vi "Operator Input Decimal.vi"(7 "Data format":string="0103ddd", 8 "error in (no error)":errorcluster, 9 "Lower limit":dbl=1.0, 10 "Upper limit":dbl=1000000000000000.0, 11 "Message":string) -> (0 "error out":errorcluster, 1 "number":i32, 2 "Stop button hit":bool, 3 "Response":string)   [LabVIEW 2013]
panel:
  in  "stop":bool
  in  "Response1":string
  # "Operator Message"
  # "Scan or Enter Response"
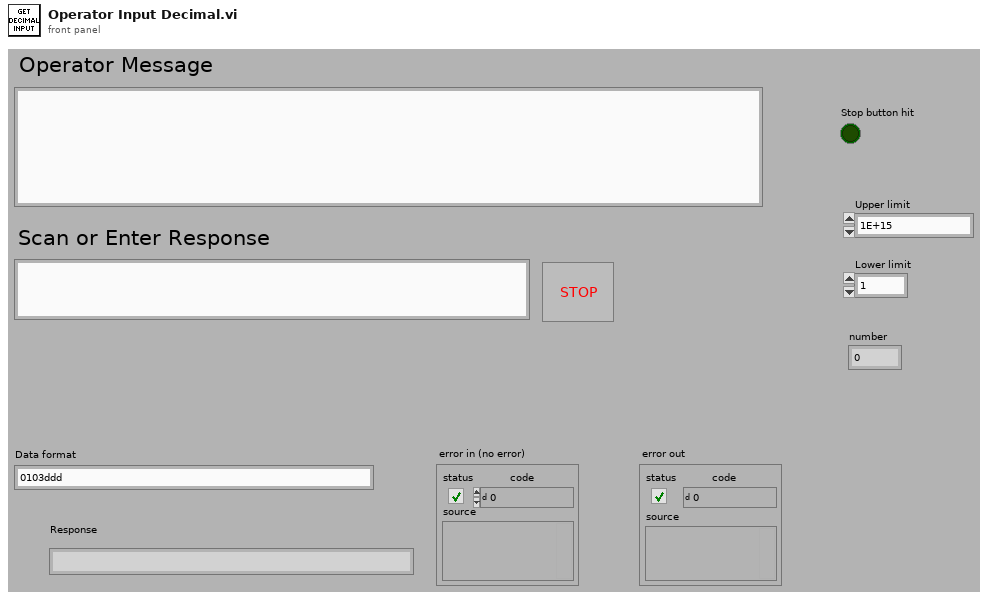
[diagram p1: front panel]
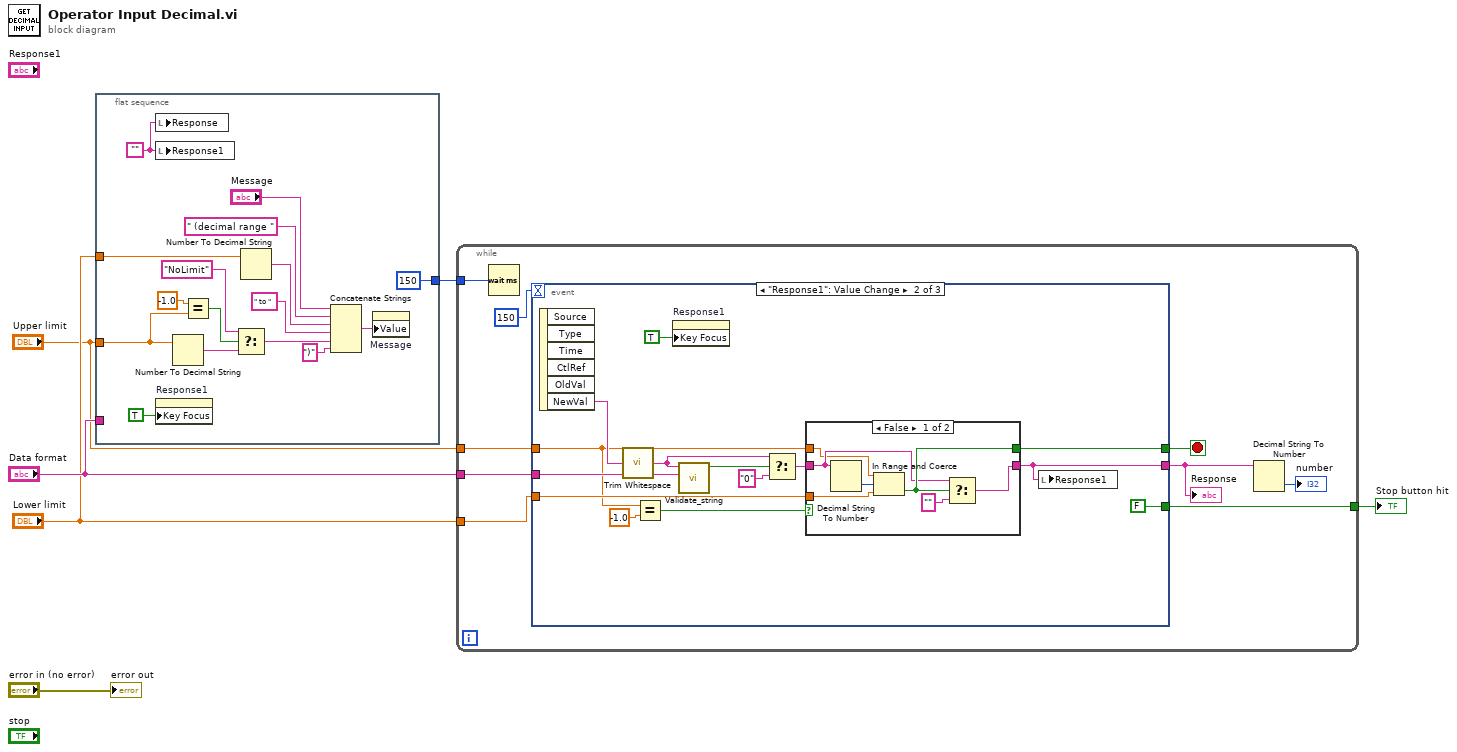
[diagram p0: block diagram]
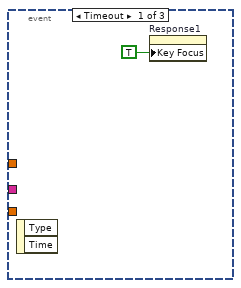
[diagram p2: hidden frame]
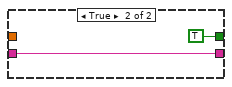
[diagram p3: hidden frame]
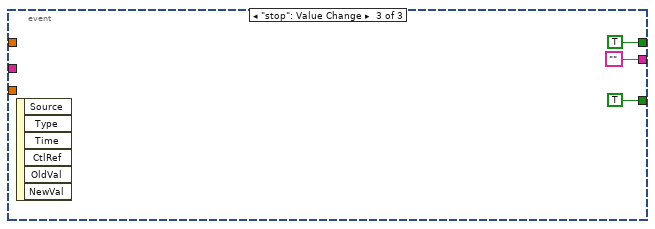
[diagram p4: hidden frame]
diagram:
  n1 = flat-sequence {
    tunnel: [u32 150 ("milliseconds to wait")] -> w6
    tunnel: "Data format" -> [_]
    tunnel: "Lower limit" -> [w16]
    tunnel: "Upper limit" -> [w12]
    frame #0 {
      w21 = ""
      n2 = local write "Response"(w21) -> ()
      n3 = local write "Response1"(w21) -> ()
      n4 = property on="Response1" class="Str"("Key Focus"=TRUE) -> ()  [unwired: 2 in, 2 out]
      n5 = Number To Decimal String(number=w12) -> (decimal integer string=w9:string)  [unwired: 1 in]
      n6 = Equal?(x=-1.0, y=w12) -> (x = y?=w10:bool)
      n7 = Select(t="NoLimit", s=w10, f=w9) -> (s? t:f=w8:string)
      n8 = Number To Decimal String(number=w16) -> (decimal integer string=w15:string)  [unwired: 1 in]
      n9 = Concatenate Strings("Message", " (decimal range " ("string"), w15, " to " ("string"), w8, ")" ("string")) -> (w17:string)
      n10 = property on="Message" class="Str"("Value"=w17) -> ()  [unwired: 2 in, 2 out]
    }
  }
  n11 = while {
    tunnel: w6 -> [w31]
    tunnel: [w29] -> w4
    tunnel: "Data format" -> [w28]
    tunnel: "Upper limit" -> [w26]
    tunnel: "Lower limit" -> [w25]
    stop <- w30 stop-if-true
    n12 = Wait (ms)(milliseconds to wait=w31) -> ()  [unwired: 1 out]
    n13 = event shown="[1] \"Response1\": Value Change" {
      selector: _ -> [_ _ _]
      dyn-events: _ -> [_ _ _]
      timeout: 150 -> [_ _ _]
      tunnel: [_ w45 TRUE] -> w30
      tunnel: [_ w44 ""] -> w24
      tunnel: [_ FALSE TRUE] -> w29
      tunnel: w28 -> [_ w37 _]
      tunnel: w26 -> [_ w35 _]
      tunnel: w25 -> [_ w36 _]
      event Timeout {
        n14 = event-data() -> ()  [unwired: 1 in, 2 out]
        n15 = property on="Response1" class="Str"("Key Focus"=TRUE) -> ()  [unwired: 2 in, 2 out]
      }
      event "Response1": Value Change {
        n16 = event-data() -> ("NewVal"=w39:string)  [unwired: 1 in, 5 out]
        n17 = call <vilib>:"Trim Whitespace.vi"("string"=w39) -> ("trimmed string"=w38:string)  [unwired: 1 in]
        n18 = Equal?(x=w35, y=-1.0 ("Upper limit")) -> (x = y?=w33:bool)
        n19 = property on="Response1" class="Str"("Key Focus"=TRUE) -> ()  [unwired: 2 in, 2 out]
        n20 = call "Validate_string.vi"("String data format"=w37, "String"=w38) -> ("String Valid"=w42:bool)  [unwired: 8 in, 1 out]
        n21 = Select(t=w38, s=w42, f="0") -> (s? t:f=w40:string)
        n22 = case shown="False" w33 {
          tunnel: [w51 TRUE] -> w45
          tunnel: [w50 w54] -> w44
          tunnel: w40 -> [w49 w54]
          tunnel: w36 -> [w48 _]
          tunnel: w35 -> [w47 _]
          frame False {
            n23 = Decimal String To Number(string=w49) -> (number=w53:i32)  [unwired: 2 in, 1 out]
            n24 = In Range and Coerce(upper limit=w47, x=w53, lower limit=w48) -> (In Range?=w51:bool)  [unwired: 1 out]
            n25 = Select(t=w49, s=w51, f="") -> (s? t:f=w50:string)
          }
          frame True {
          }
        }
        n26 = local write "Response1"(w44) -> ()
      }
      event "stop": Value Change {
        n27 = event-data() -> ()  [unwired: 1 in, 6 out]
      }
    }
    "Response" <- w24
    n28 = Decimal String To Number(string=w24) -> (number=→"number":i32)  [unwired: 2 in, 1 out]
  }
  "Stop button hit" <- w4
  "error out" <- "error in (no error)"
